vi "Sub_Cursor_Control.vi"(8 "Range":dbl, 9 "XY 그래프":refnum<vi>, 10 "CursRef":refnum<vi>, 11 "Cursor Mode":enum16{"Free", "Sample"}(ring)) -> ()   [LabVIEW 2015]
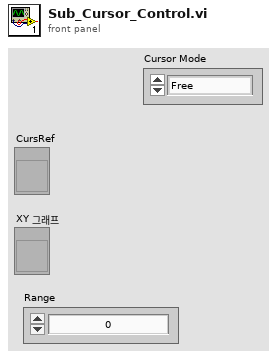
[diagram p1: front panel]
types:
  T1 = typedef "LVCursorListTypeDef.ctl" = cluster{"Name":string, "Color":u32, "Style":u8, "Point Style":u8, "Name Visible":bool, "Allow Drag":bool, "Cursor Mode":u32, "Plot":i32, "Index":i32, "Position":cluster{"X":dbl, "Y":dbl}, "X Scale":u32, "Y Scale":u32, "Watch Plots":i32[], "Watch All Plots":bool, "Plot Area":i32, "Label Offset":cluster{"X":dbl, "Y":dbl}}[]
  T2 = cluster{"Name":string, "Color":u32, "Style":u8, "Point Style":u8, "Name Visible":bool, "Allow Drag":bool, "Cursor Mode":u32, "Plot":i32, "Index":i32, "Position":cluster{"X":dbl, "Y":dbl}, "X Scale":u32, "Y Scale":u32, "Watch Plots":i32[], "Watch All Plots":bool, "Plot Area":i32, "Label Offset":cluster{"X":dbl, "Y":dbl}}
  T3 = cluster{"Name":string, "Color":u32, "Style":u8, "Point Style":u8, "Name Visible":bool, "Allow Drag":bool, "Cursor Mode":u32, "Plot":i32, "Index":i32, "Position":cluster{"X":dbl, "Y":dbl}, "X Scale":u32, "Y Scale":u32, "Watch Plots":i32[], "Watch All Plots":bool, "Plot Area":i32, "Label Offset":cluster{"X":dbl, "Y":dbl}}[]
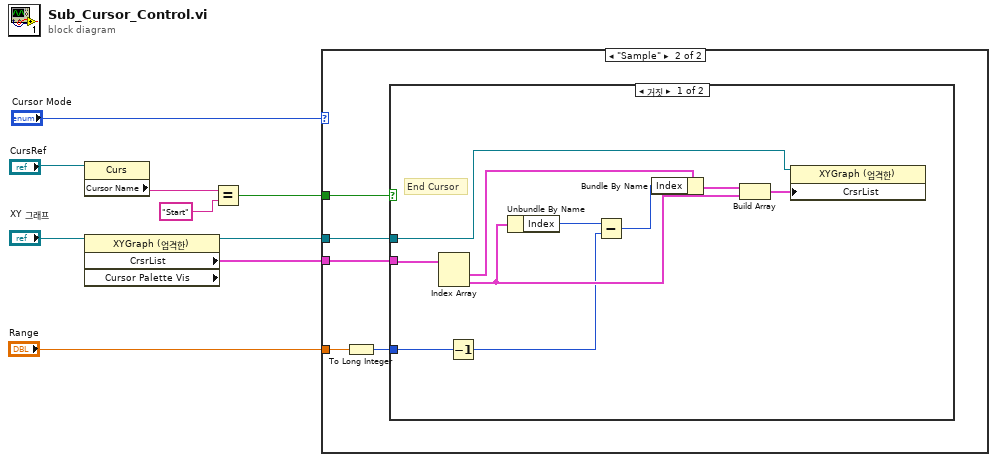
[diagram p0: block diagram]
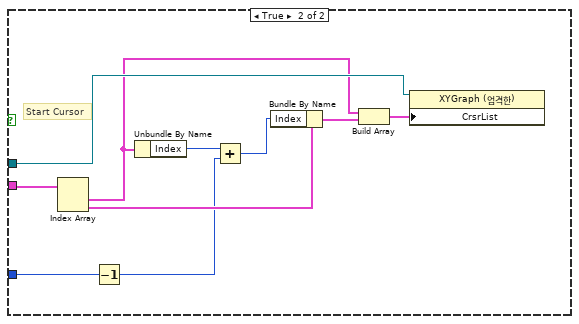
[diagram p3: hidden frame]
diagram:
  n1 = property class="Curs"(reference="CursRef") -> ("Cursor Name"=w3:string)  [unwired: 1 in, 2 out]
  n2 = property class="XYGraph (엄격한)" props=["CrsrList", "Cursor Palette Vis"](reference="XY 그래프") -> (reference out=w6:refnum<vi>, "CrsrList"=w7:T1)  [unwired: 1 in, 2 out]
  n3 = Equal?(x=w3, y="Start") -> (x = y?=w2:bool)
  n4 = case shown="\"Sample\"" "Cursor Mode" {
    tunnel: w7 -> [_ w14]
    tunnel: w6 -> [_ w13]
    tunnel: w2 -> [_ w12]
    tunnel: "Range" -> [_ w11]
    frame "Free", Default {
    }
    frame "Sample" {
      n5 = To Long Integer(number=w11) -> (32bit integer=w10:i32)
      n6 = case shown="거짓" w12 {
        tunnel: w14 -> [w24 w34]
        tunnel: w13 -> [w19 w31]
        tunnel: w10 -> [w22 w33]
        frame False {
          # "End Cursor"
          n7 = Index Array(array=w24) -> (element #1=w23:T2, element #2=w20:T2)  [unwired: 2 in]
          n8 = Decrement(x=w22) -> (x-1=w15:i32)
          n9 = Unbundle By Name(w20) -> ("Index"=w16:i32)
          n10 = Subtract(x=w16, y=w15) -> (x-y=w17:i32)
          n11 = Bundle By Name(cluster=w23, "Index"=w17) -> (w21:T2)
          n12 = Build Array(w21, w20) -> (w18:T3)
          n13 = property class="XYGraph (엄격한)"(reference=w19, "CrsrList"=w18) -> ()  [unwired: 1 in, 2 out]
        }
        frame True {
          # "Start Cursor"
          n14 = Index Array(array=w34) -> (element #1=w28:T2, element #2=w29:T2)  [unwired: 2 in]
          n15 = Decrement(x=w33) -> (x-1=w25:i32)
          n16 = Unbundle By Name(w28) -> ("Index"=w26:i32)
          n17 = Add(x=w26, y=w25) -> (x+y=w32:i32)
          n18 = Bundle By Name(cluster=w29, "Index"=w32) -> (w27:T2)
          n19 = Build Array(w28, w27) -> (w30:T3)
          n20 = property class="XYGraph (엄격한)"(reference=w31, "CrsrList"=w30) -> ()  [unwired: 1 in, 2 out]
        }
      }
    }
  }
